vi "Handler - Check for Data.vi"(8 "error in (no error)":errorcluster, 11 "File IO Data in":T1={"Testing State"=FALSE, "Recording State"=FALSE, "TDMS File Ref"=refnum, "APU Setup File Ref"=refnum, "App Data Directory"=path "", "Data Directory"=path "", "APU Setup Filepath"=path "", "APU Select"="<Select>", "Test Information"={"APU Part Number:"="", "Model:"="", "Serial Number:"="", "Customer:"="", "Work Order:"="", "Repair Level:"=""}, "Crash Log Data"=[], "Group Name"="", "APU Setup File"={"Sensor Info"=[], "Calibration Info"=[], "CMM Table 106"=[], "CMM Table 106B "=[], "Report Helper"=[]}, "Work Order Path"=path "", "Report path"=path "", "Report Template Path"=path "", "APURunCount"=0}) -> (0 "error out":errorcluster, 3 "File IO Data out":T1={"Testing State"=FALSE, "Recording State"=FALSE, "TDMS File Ref"=refnum, "APU Setup File Ref"=refnum, "App Data Directory"=path "", "Data Directory"=path "", "APU Setup Filepath"=path "", "APU Select"="<Select>", "Test Information"={"APU Part Number:"="", "Model:"="", "Serial Number:"="", "Customer:"="", "Work Order:"="", "Repair Level:"=""}, "Crash Log Data"=[], "Group Name"="", "APU Setup File"={"Sensor Info"=[], "Calibration Info"=[], "CMM Table 106"=[], "CMM Table 106B "=[], "Report Helper"=[]}, "Work Order Path"=path "", "Report path"=path "", "Report Template Path"=path "", "APURunCount"=0})   [LabVIEW 2018]
doc: "Responsible for the data buffer and dumping the data into a TMDS file."
uses:
  File IO.lvlib
  Top Level/Shared Controls/Analyzed Data Sets.ctl
  Top Level/Shared Controls/All Data Cluster.ctl
  Top Level/Shared Controls/Acq Data.ctl
  Top Level/Shared Controls/Post-Analysis Data.ctl
  Top Level/Shared Controls/Calculated Data.ctl
  Controller (Host)/Public Controls/Test Information.ctl
  Controller (Host)/Controller (Host).lvlib
  Private Controls/File IO Data.ctl
  Controller (Host)/Public Controls/APU Select.ctl
  Top Level/Shared Controls/APU Setup File.ctl
panel:
  # "Test Information:"
  # "Test Information:"
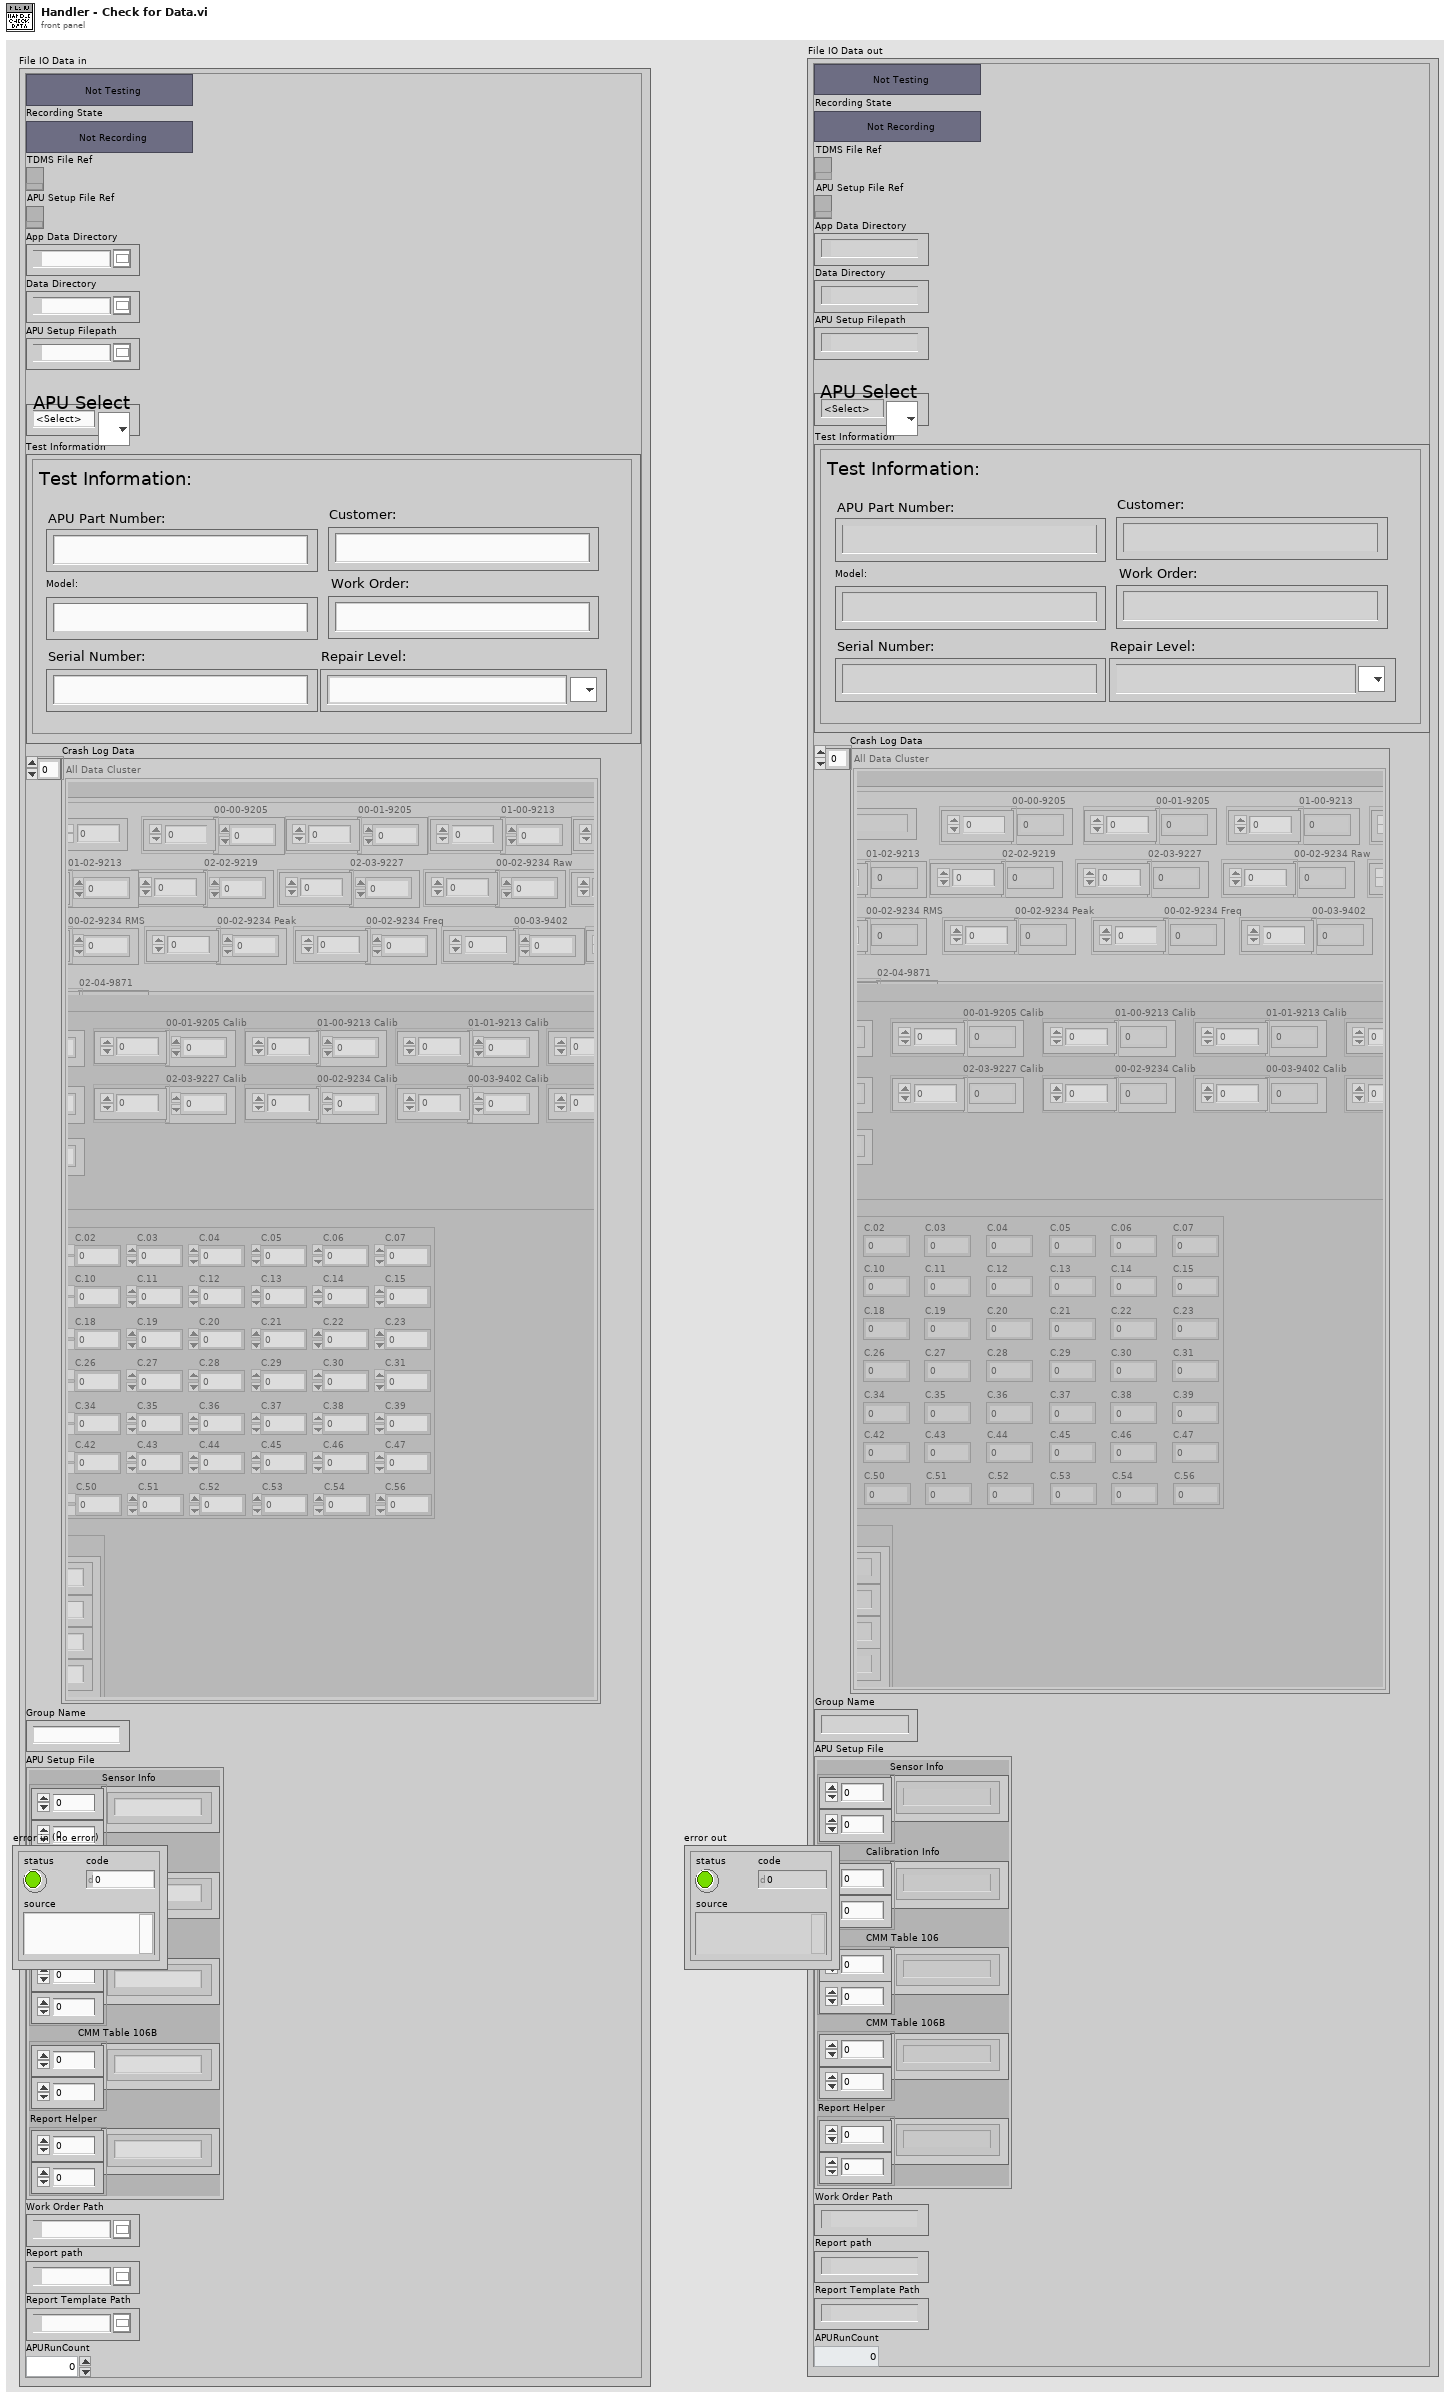
[diagram p1: front panel]
types:
  T1 = typedef "File IO.lvlib/File IO Data.ctl" = cluster{"Testing State":bool, "Recording State":bool, "TDMS File Ref":refnum<k34>, "APU Setup File Ref":refnum<k34>, "App Data Directory":path, "Data Directory":path, "APU Setup Filepath":path, "APU Select":T2, "Test Information":T3, "Crash Log Data":T4, "Group Name":string, "APU Setup File":T9, "Work Order Path":path, "Report path":path, "Report Template Path":path, "APURunCount":u32}
  T2 = typedef "Controller (Host).lvlib/APU Select.ctl" = string
  T3 = typedef "Controller (Host).lvlib/Test Information.ctl" = cluster{"APU Part Number:":string, "Model:":string, "Serial Number:":string, "Customer:":string, "Work Order:":string, "Repair Level:":string}
  T4 = typedef "Analyzed Data Sets.ctl" = T5[]
  T5 = typedef "All Data Cluster.ctl" = cluster{"Acq Data":T6, "Post-Analysis Data":T7}
  T6 = typedef "Acq Data.ctl" = cluster{"Timestamp":timestamp, "Acq Period (ms)":i64, "00-00-9205":dbl[], "00-01-9205":dbl[], "01-00-9213":dbl[], "01-01-9213":dbl[], "01-02-9213":dbl[], "02-02-9219":dbl[], "02-03-9227":dbl[], "00-02-9234 Raw":dbl[], "00-02-9234 DC":dbl[], "00-02-9234 RMS":dbl[], "00-02-9234 Peak":dbl[], "00-02-9234 Freq":dbl[], "00-03-9402":dbl[], "02-05-9205":dbl[], "02-04-9871":dbl[]}
  T7 = typedef "Post-Analysis Data.ctl" = cluster{"Calibrated Data":cluster{"00-00-9205 Calib":dbl[], "00-01-9205 Calib":dbl[], "01-00-9213 Calib":dbl[], "01-01-9213 Calib":dbl[], "01-02-9213 Calib":dbl[], "02-02-9219 Calib":dbl[], "02-03-9227 Calib":dbl[], "00-02-9234 Calib":dbl[], "00-03-9402 Calib":dbl[], "02-05-9205 Calib":dbl[], "02-04-9871 2DArray":dbl[][]}, "Calculated Data":T8, "Indicator Data":cluster{"00-02-9234 Peak Vel (in/sec)":dbl[]}}
  T8 = typedef "Calculated Data.ctl" = cluster{"C.00":dbl, "C.01":dbl, "C.02":dbl, "C.03":dbl, "C.04":dbl, "C.05":dbl, "C.06":dbl, "C.07":dbl, "C.08":dbl, "C.09":dbl, "C.10":dbl, "C.11":dbl, "C.12":dbl, "C.13":dbl, "C.14":dbl, "C.15":dbl, "C.16":dbl, "C.17":dbl, "C.18":dbl, "C.19":dbl, "C.20":dbl, "C.21":dbl, "C.22":dbl, "C.23":dbl, "C.24":dbl, "C.25":dbl, "C.26":dbl, "C.27":dbl, "C.28":dbl, "C.29":dbl, "C.30":dbl, "C.31":dbl, "C.32":dbl, "C.33":dbl, "C.34":dbl, "C.35":dbl, "C.36":dbl, "C.37":dbl, "C.38":dbl, "C.39":dbl, "C.40":dbl, "C.41":dbl, "C.42":dbl, "C.43":dbl, "C.44":dbl, "C.45":dbl, "C.46":dbl, "C.47":dbl, "C.48":dbl, "C.49":dbl, "C.50":dbl, "C.51":dbl, "C.52":dbl, "C.53":dbl, "C.54":dbl, "C.56":dbl}
  T9 = typedef "APU Setup File.ctl" = cluster{"Sensor Info":string[][], "Calibration Info":string[][], "CMM Table 106":string[][], "CMM Table 106B ":string[][], "Report Helper":string[][]}
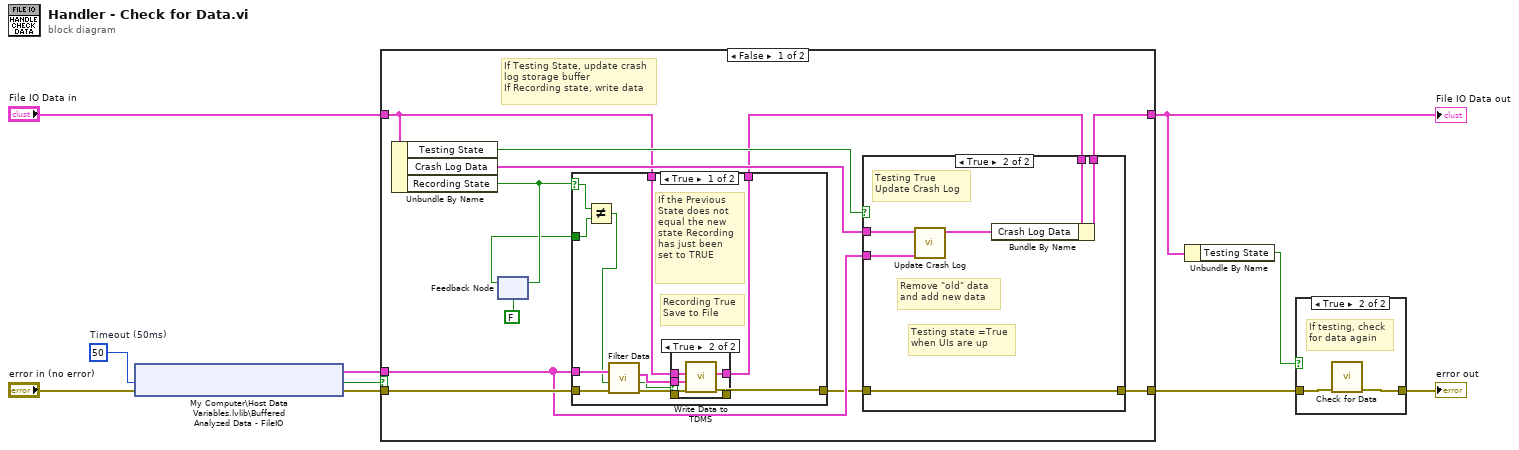
[diagram p0: block diagram]
diagram:
  w2 = 50  # Timeout (50ms)
  n1 = shared-variable "My Computer\\Host Data Variables.lvlib\\Buffered Analyzed Data - FileIO"(error in="error in (no error)", w2) -> (w5:T4, error out=w3:errorcluster, w1:bool)
  n2 = case shown="False" w1 {
    tunnel: w3 -> [w22 w52]
    tunnel: [w15 w52] -> w7
    tunnel: w5 -> [w20 _]
    tunnel: "File IO Data in" -> [w14 w51]
    tunnel: [w17 w51] -> w10
    frame False {
      # "If Testing State, update crash\nlog storage buffer\nIf Recording state, write data"
      n3 = Unbundle By Name(w14) -> ("Testing State"=w21:bool, "Crash Log Data"=w19:T4, "Recording State"=w13:bool)
      n4 = feedback-in #1(w13) -> ()
      n5 = feedback #1(FALSE ("Recording State")) -> (w12:bool)
      n6 = case shown="True" w13 {
        selector: w13 -> [w32 _]
        tunnel: [w37 w49] -> w18
        tunnel: w22 -> [w40 w50]
        tunnel: [w36 w50] -> w16
        tunnel: w20 -> [w41 _]
        tunnel: w14 -> [w38 w49]
        tunnel: w12 -> [w33 _]
        frame True {
          # "If the Previous\nState does not \nequal the new \nstate Recording \nhas just been\nset to TRUE"
          # "Recording True\nSave to File"
          n7 = Not Equal?(x=w32, y=w33) -> (x != y?=w31:bool)
          n8 = call "Filter Data.vi"("error in"=w40, "Record state change"=w31, "Analyzed Data Sets"=w41) -> ("error out"=w39:errorcluster, "Send?"=w34:bool, "Analyzed Data Sets Out"=w35:T4)  [unwired: 6 in]
          n9 = case shown="True" w34 {
            tunnel: w39 -> [w42 w48]
            tunnel: w38 -> [w43 w47]
            tunnel: [w43 w46] -> w37
            tunnel: [w42 w45] -> w36
            tunnel: w35 -> [_ w44]
            frame False {
            }
            frame True {
              n10 = call "Write Data to TDMS.vi"("error in"=w48, "Data"=w44, "File IO Data In"=w47) -> ("error out"=w45:errorcluster, "File IO Data Out"=w46:T1)  [unwired: 6 in, 1 out]
            }
          }
        }
        frame False {
        }
      }
      n11 = case shown="True" w21 {
        tunnel: w20 -> [_ w25]
        tunnel: w19 -> [_ w27]
        tunnel: w18 -> [w23 w30]
        tunnel: [w23 w29] -> w17
        tunnel: w16 -> [w24 w28]
        tunnel: [w24 w28] -> w15
        frame False {
        }
        frame True {
          # "Testing state =True \nwhen UIs are up"
          # "Testing True\nUpdate Crash Log"
          # "Remove \"old\" data\nand add new data"
          n12 = call "Update Crash Log.vi"("New Crash Log Data"=w25, "Old Crash Log Data"=w27) -> ("Updated Crash Log Data"=w26:T4)  [unwired: 9 in]
          n13 = Bundle By Name(cluster=w30, "Crash Log Data"=w26) -> (w29:T1)
        }
      }
    }
    frame True {
      # "Timed out, don't do anything"
    }
  }
  "File IO Data out" <- w10
  n14 = Unbundle By Name(w10) -> ("Testing State"=w8:bool)
  n15 = case shown="True" w8 {
    tunnel: w7 -> [w53 w55]
    tunnel: [w53 w54] -> w6
    frame False {
    }
    frame True {
      # "If testing, check\nfor data again"
      n16 = call "Check for Data.vi"("error in (no error)"=w55) -> ("error out"=w54:errorcluster)  [unwired: 10 in]
    }
  }
  "error out" <- w6
